vi "생산자소비자(상태머신)-수정.vi"() -> ()   [LabVIEW 2014]
uses:
  <vilib>/Analysis/NI_AALBase.lvlib
panel:
  in  "긴급":bool
  in  "삼각파":bool
  out "웨이브폼 그래프":dbl[](graph)
  in  "사인파":bool
  in  "정지":bool
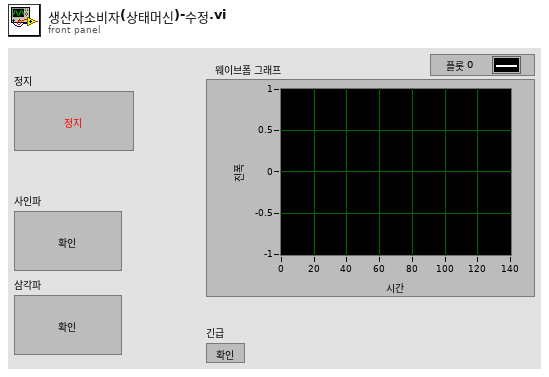
[diagram p1: front panel]
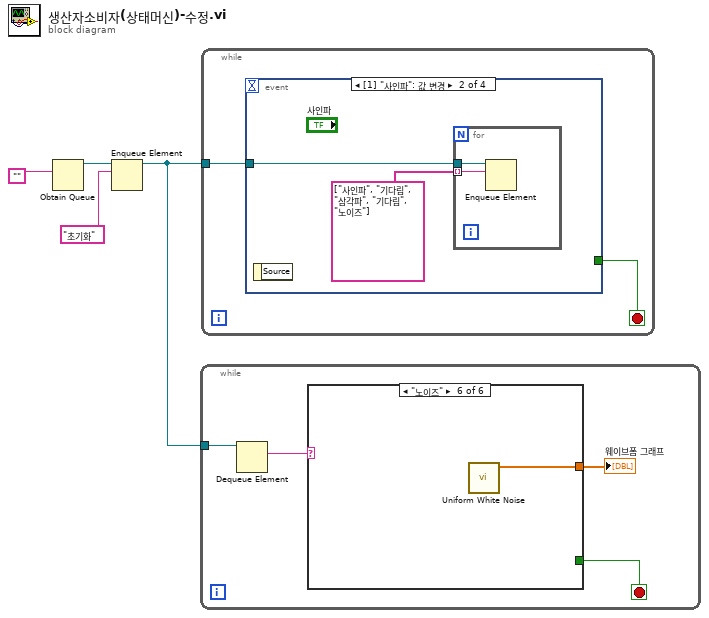
[diagram p0: block diagram]
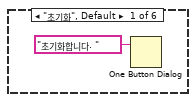
[diagram p2: hidden frame]
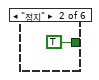
[diagram p3: hidden frame]
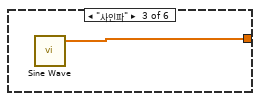
[diagram p4: hidden frame]
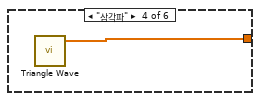
[diagram p5: hidden frame]
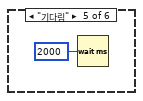
[diagram p6: hidden frame]
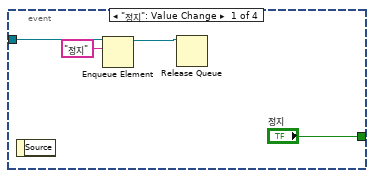
[diagram p7: hidden frame]
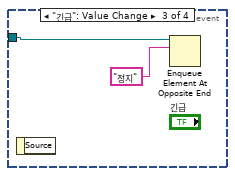
[diagram p8: hidden frame]
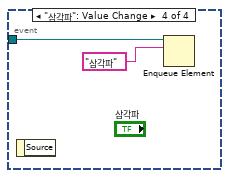
[diagram p9: hidden frame]
diagram:
  n1 = Obtain Queue(element data type="") -> (queue out=w4:refnum<queue>)  [unwired: 4 in, 2 out]
  n2 = Enqueue Element(queue=w4, element="초기화" ("원소")) -> (queue out=w3:refnum<queue>)  [unwired: 2 in, 2 out]
  n3 = while {
    tunnel: w3 -> [w8]
    stop <- w7 stop-if-true
    n4 = Dequeue Element(queue=w8) -> (element=w5:string)  [unwired: 2 in, 3 out]
    n5 = case shown="\"노이즈\"" w5 {
      tunnel: [_ TRUE _ _ _ _] -> w7
      tunnel: [_ _ w11 w12 _ w14] -> w6
      frame "초기화", Default {
        n6 = One Button Dialog(message="초기화합니다. " ("메시지")) -> ()  [unwired: 1 in, 1 out]
      }
      frame "정지" {
      }
      frame "사인파" {
        n7 = call <vilib>:"Sine Wave.vi"() -> ("sine wave"=w11:dbl[])  [unwired: 5 in, 2 out]
      }
      frame "삼각파" {
        n8 = call <vilib>:"Triangle Wave.vi"() -> ("triangle wave"=w12:dbl[])  [unwired: 5 in, 2 out]
      }
      frame "기다림" {
        n9 = Wait (ms)(milliseconds to wait=u32 2000 ("대기 시간(ms)")) -> ()  [unwired: 1 out]
      }
      frame "노이즈" {
        n10 = call <vilib>:"Uniform White Noise.vi"() -> ("uniform white noise"=w14:dbl[])  [unwired: 10 in, 1 out]
      }
    }
    "웨이브폼 그래프" <- w6
  }
  n11 = while {
    tunnel: w3 -> [w16]
    stop <- w15 stop-if-true
    n12 = event shown="[1] \"사인파\": 값 변경" {
      selector: _ -> [_ _ _ _]
      dyn-events: _ -> [_ _ _ _]
      timeout: _ -> [_ _ _ _]
      tunnel: w16 -> [w19 w22 w26 w28]
      tunnel: ["정지" _ _ _] -> w15
      event "정지": Value Change {
        n13 = event-data() -> ()  [unwired: 1 in, 1 out]
        n14 = Enqueue Element(queue=w19, element="정지" ("원소")) -> (queue out=w18:refnum<queue>)  [unwired: 2 in, 2 out]
        n15 = Release Queue(queue=w18) -> ()  [unwired: 2 in, 3 out]
      }
      event "사인파": Value Change {
        n16 = event-data() -> ()  [unwired: 1 in, 1 out]
        n17 = for {
          tunnel: w22 -> [w24]
          tunnel: string[] ["사인파", "기다림", "삼각파", "기다림", "노이즈"] -> [w23] mode=indexing
          n18 = Enqueue Element(queue=w24, element=w23) -> ()  [unwired: 2 in, 3 out]
        }
      }
      event "긴급": Value Change {
        n19 = event-data() -> ()  [unwired: 1 in, 1 out]
        n20 = Enqueue Element At Opposite End(queue=w26, element="정지" ("원소")) -> ()  [unwired: 2 in, 3 out]
      }
      event "삼각파": Value Change {
        n21 = event-data() -> ()  [unwired: 1 in, 1 out]
        n22 = Enqueue Element(queue=w28, element="삼각파" ("원소")) -> ()  [unwired: 2 in, 3 out]
      }
    }
  }
